vi "EBA Leak test.vi"() -> ()   [LabVIEW 2025]
uses:
  Control EBA.ctl
panel:
  out "Current int":i32
  out "Exit - Entry":i32
  out "Entry int":i32
  out "Exit":i32
  in  "Tab Control":enum32{"Page 1", "Page 2"}(tab)
  out "Checkbox":bool
  out "Save Status":string
  out "Leak rate cc/min":dbl format="%.2f"
  out "Pressure vs Time":dynamicdata(graph)
  out "Info":string
  in  "Stop":bool
  in  "Start":bool
  out "Initial Pressure (Bar)":dbl format="%.3f"
  in  "File Location":path=path "C:/Users/G MOHANASUNDAR/OneDrive/Desktop/Project_EBA/Raw Data/Leak.xlsx" caption="Filename"
  out "Hold Time (s)":dbl format="%.2g"
  out "Current Pressure (Bar)":dbl format="%.2f"
  out "Final Pressure (Bar)":dbl format="%.2f"
  out "error out":errorcluster
  in  "Hold time (s)":dbl=60.0 format="%#_13g"
  # "EBA LEAK THROUGH PUSH TEST"
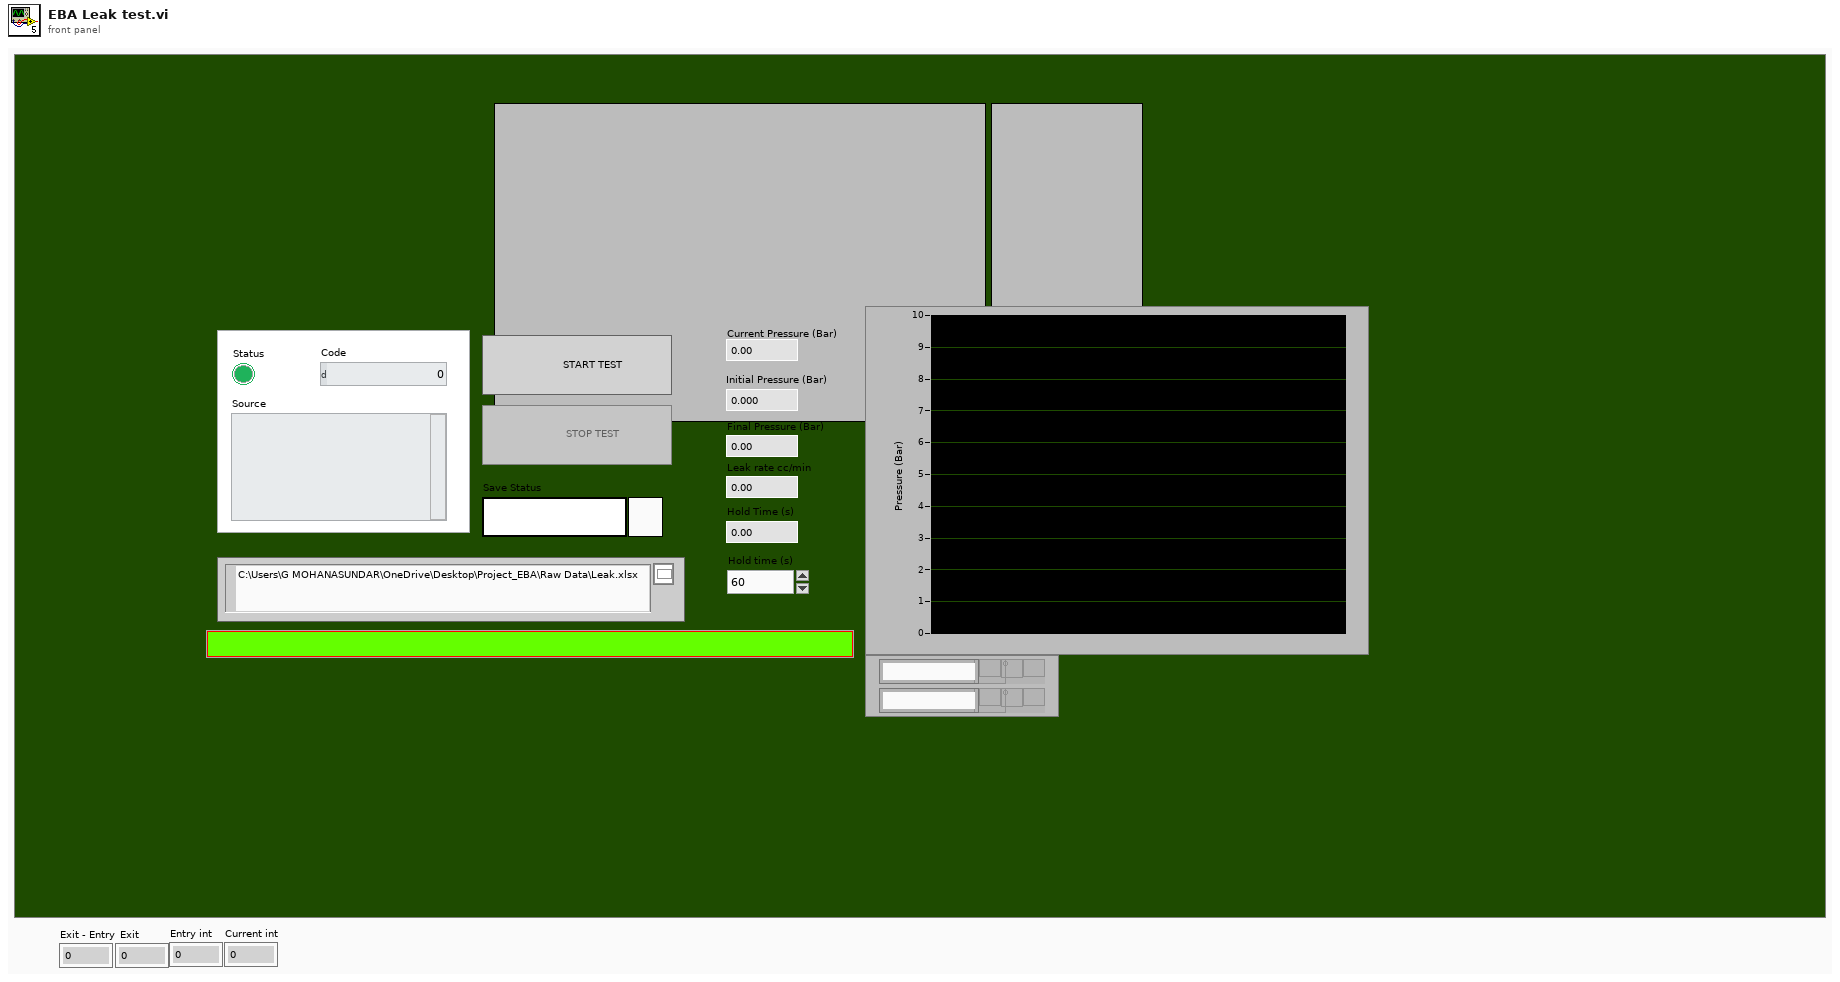
[diagram p1: front panel]
types:
  T1 = typedef "Control EBA.ctl" = enum16{"Wait for event", "Running", "Log", "Stopped", "Leak check", "Calc", "Login", "Update"}
  T2 = cluster{"True?":bool, "time":dbl, "pressure":dbl}
  T3 = enum8{"Enabled", "Disabled", "Disabled and Grayed Out"}
  T4 = enum16{"Wait for event", "Running", "Log", "Stopped"}
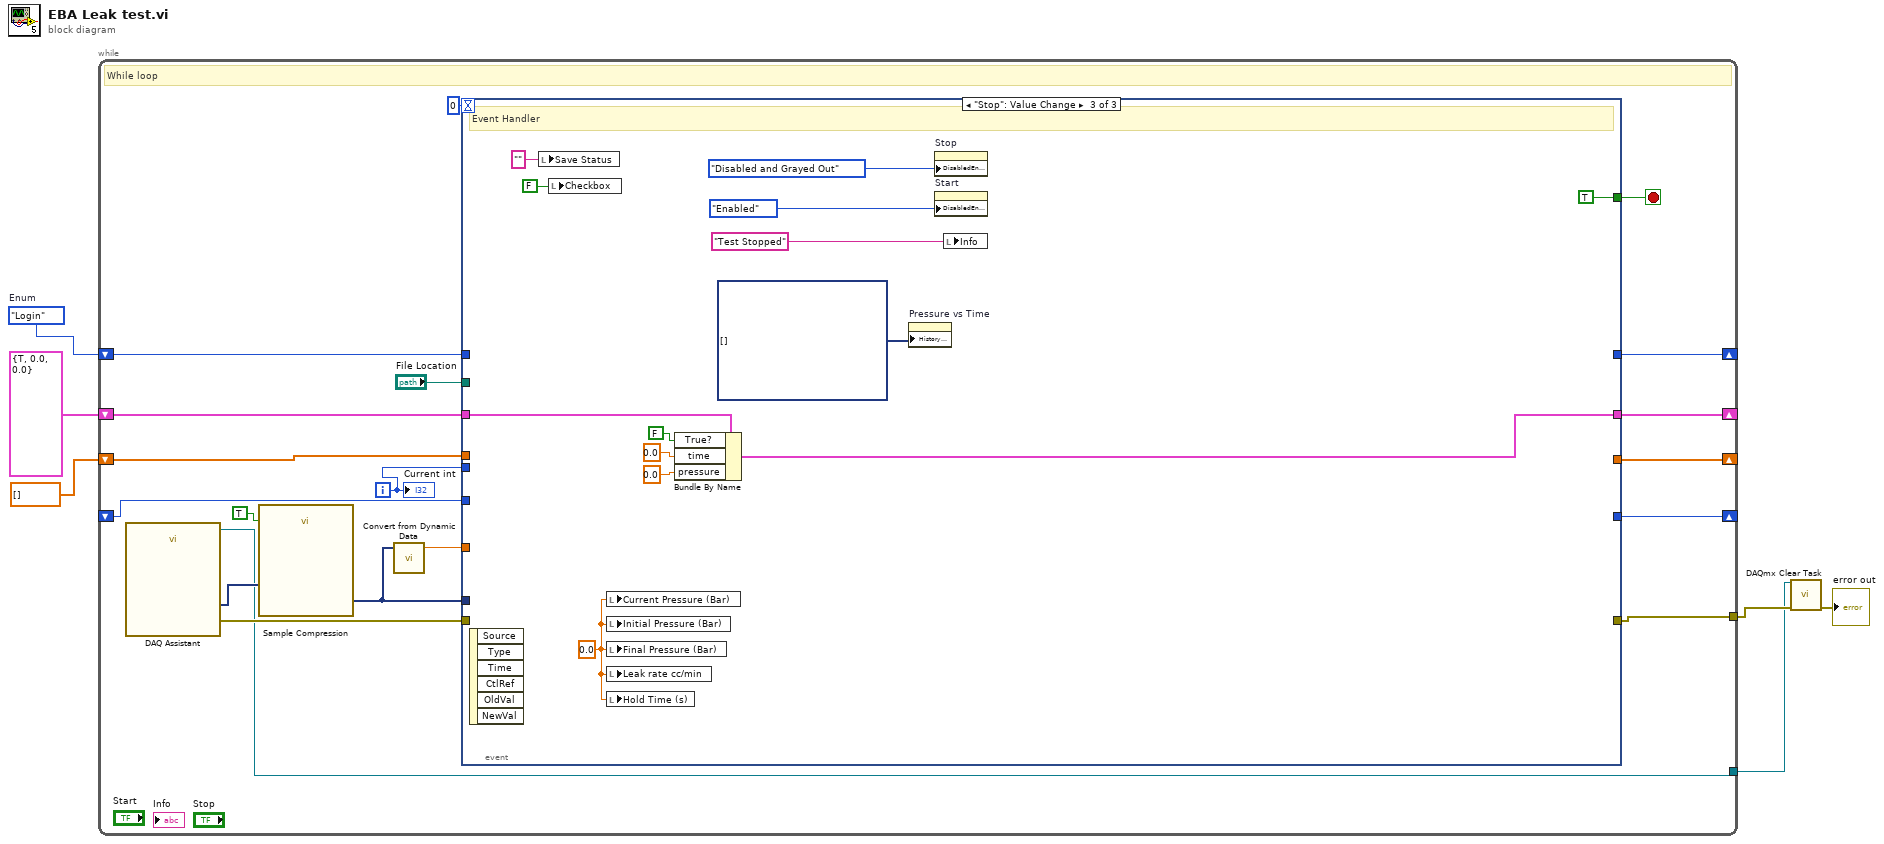
[diagram p0: block diagram]
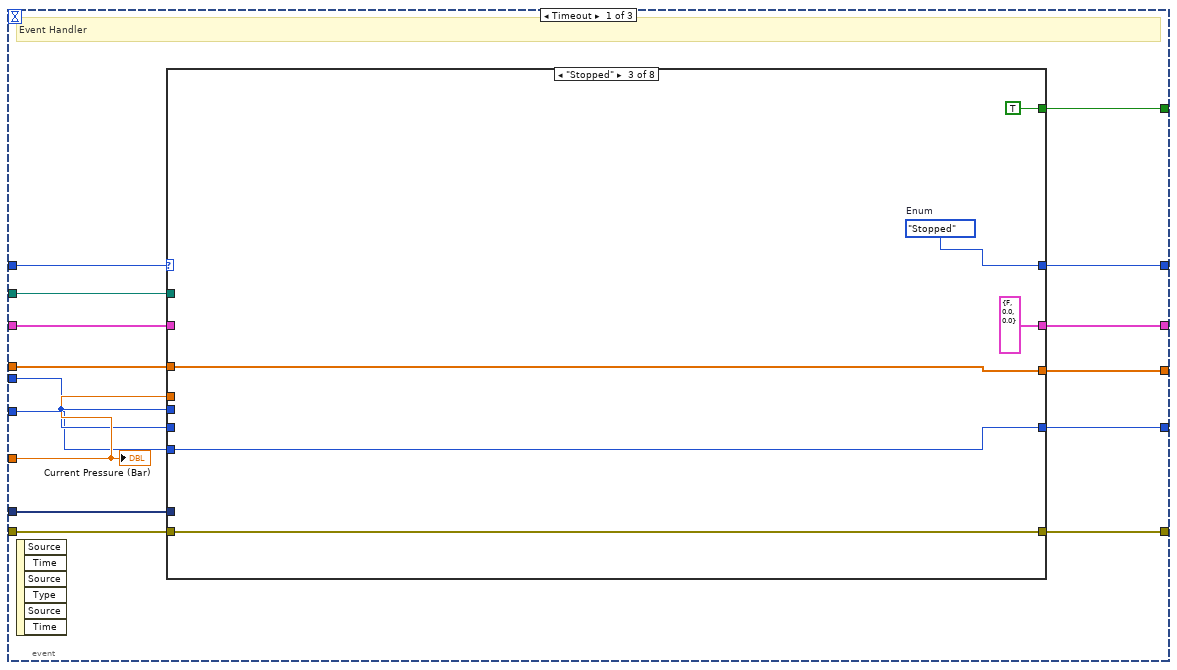
[diagram p2: hidden frame]
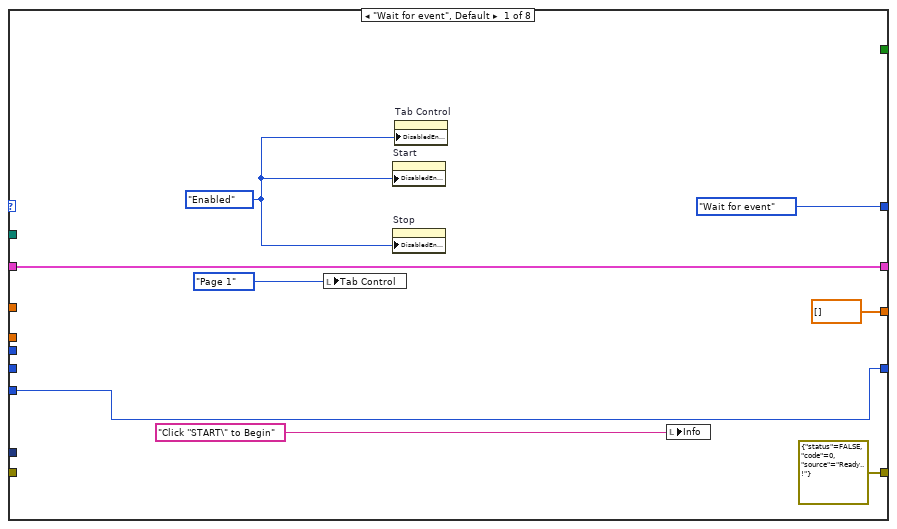
[diagram p3: hidden frame]
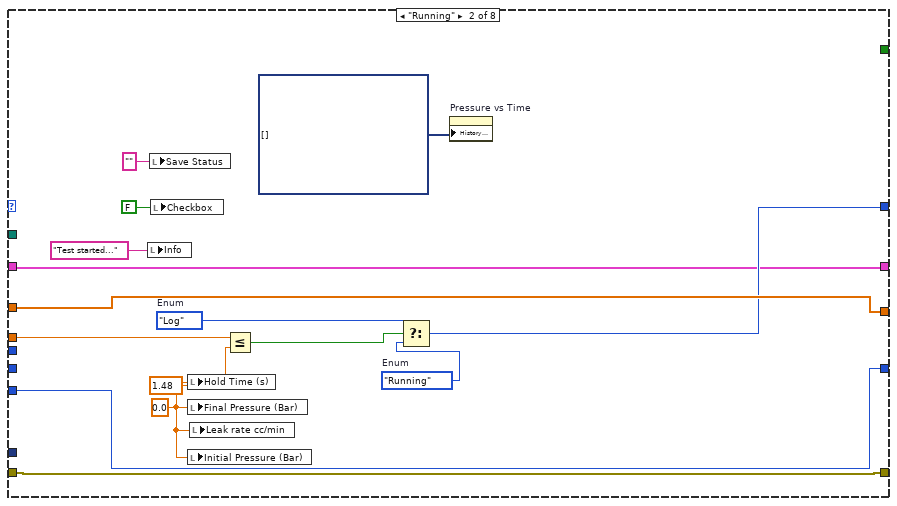
[diagram p4: hidden frame]
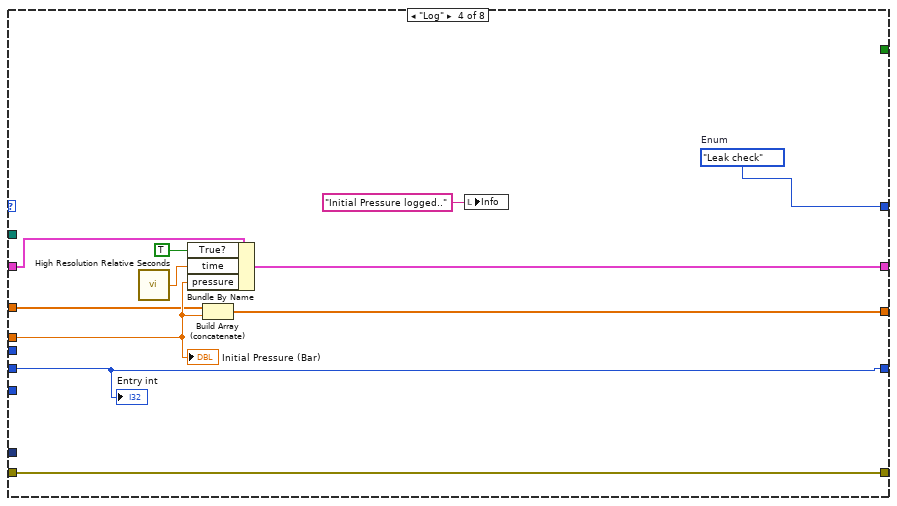
[diagram p5: hidden frame]
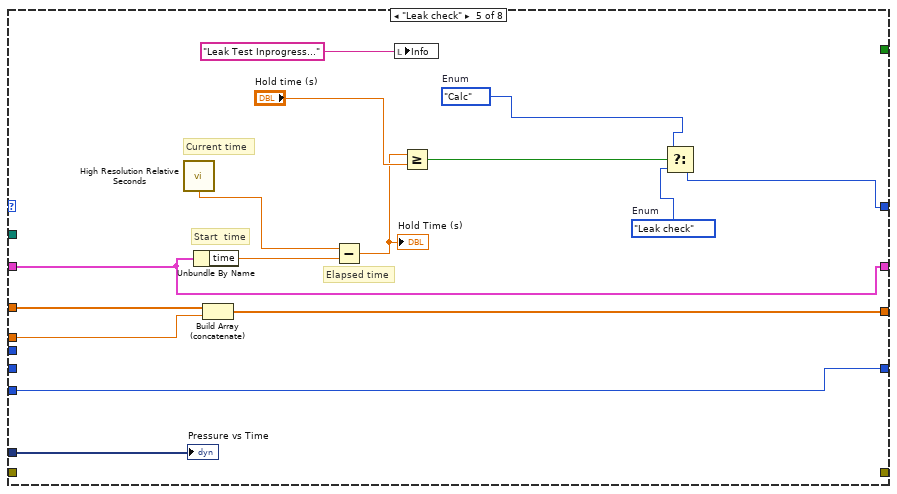
[diagram p6: hidden frame]
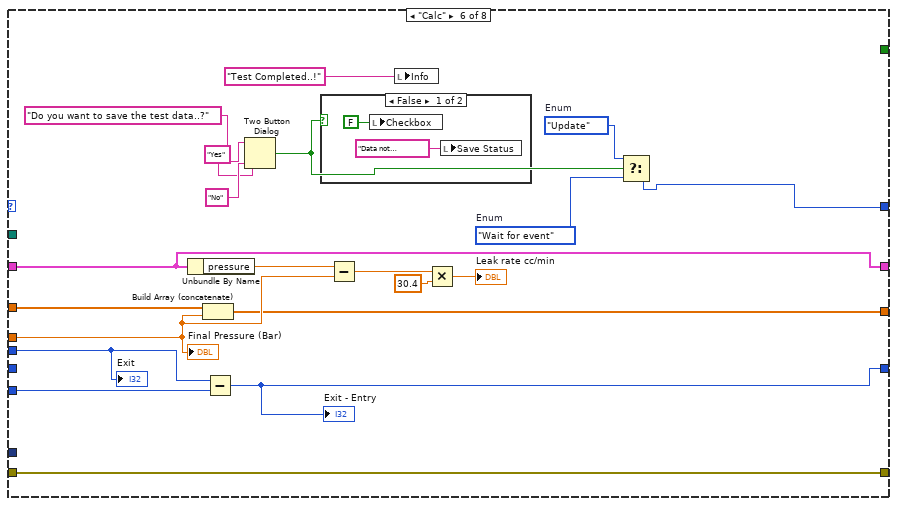
[diagram p7: hidden frame]
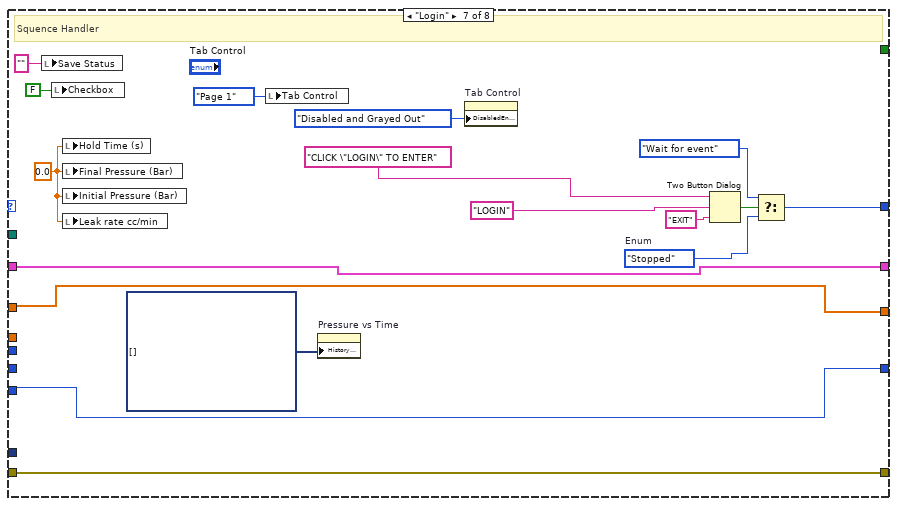
[diagram p9: hidden frame]
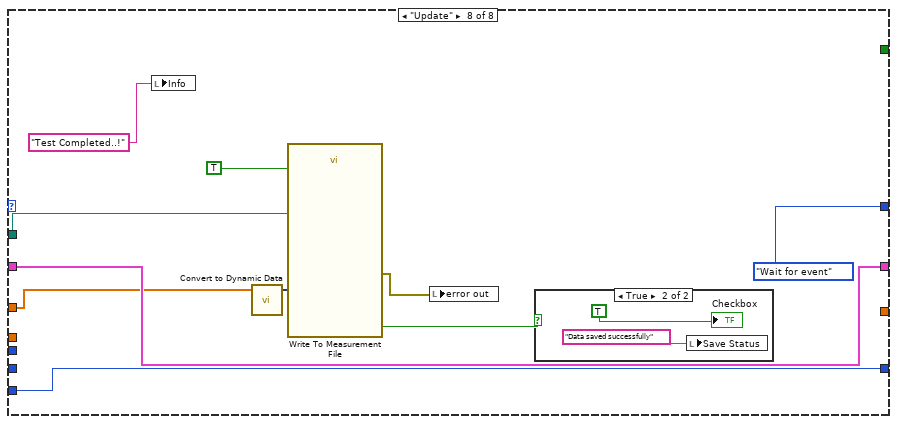
[diagram p10: hidden frame]
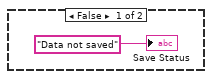
[diagram p11: hidden frame]
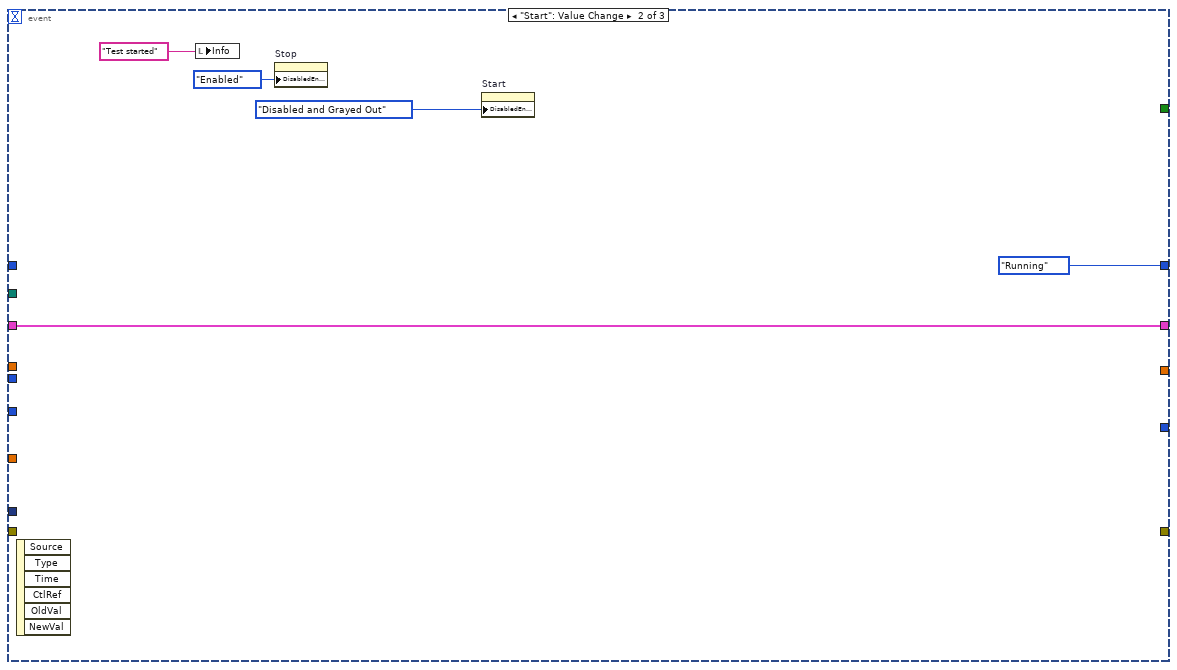
[diagram p12: hidden frame]
diagram:
  w4 = Control_EBA."Login"  # Enum
  n1 = while {
    shift-right: [w23] -> _
    shift-left: T2 {"True?"=TRUE, "time"=0.0, "pressure"=0.0} -> [w24]
    shift-right: [w15] -> _
    shift-left: _ -> [w14]
    shift-right: [w12] -> _
    shift-left: dbl[] [] -> [w13]
    shift-right: [w10] -> _
    shift-left: w4 -> [w25]
    tunnel: [w8] -> w3
    tunnel: [w7] -> w1
    i -> [w16]
    stop <- w22 stop-if-true
    # "While loop"
    n2 = call "DAQ Assistant"() -> ("task out"=w7:refnum<k21>, "data"=w19:dynamicdata, "error out"=w20:errorcluster)  [unwired: 16 in, 1 out]
    n3 = call "Sample Compression"("Enable"=TRUE, "Signals"=w19) -> ("Mean"=w18:dynamicdata)  [unwired: 7 in, 2 out]
    n4 = call "Convert from Dynamic Data"("Dynamic Data Type"=w18) -> ("Scalar"=w21:dbl)  [unwired: 3 in]
    n5 = event shown="[2] \"Stop\": Value Change" {
      selector: _ -> [_ _ _]
      dyn-events: _ -> [_ _ _]
      timeout: 0 -> [_ _ _]
      tunnel: w25 -> [w40 _ _]
      tunnel: w24 -> [w39 w151 w164]
      tunnel: [w38 w151 w163] -> w23
      tunnel: [w27 T4."Running" _] -> w10
      tunnel: [w37 _ TRUE] -> w22
      tunnel: w21 -> [w33 _ _]
      tunnel: [w36 _ _] -> w8
      tunnel: w20 -> [w35 _ _]
      tunnel: w18 -> [w34 _ _]
      tunnel: w16 -> [w31 _ _]
      tunnel: [w32 _ _] -> w15
      tunnel: w14 -> [w30 _ _]
      tunnel: w13 -> [w29 _ _]
      tunnel: [w28 _ _] -> w12
      tunnel: "File Location" -> [w26 _ _]
      event Timeout {
        # "Event Handler"
        n6 = event-data() -> ()  [unwired: 1 in, 6 out]
        n7 = case shown="\"Stopped\"" w40 {
          tunnel: w39 -> [w48 w52 _ w80 w93 w112 w129 w140]
          tunnel: w33 -> [_ w63 _ w72 w84 w105 _ _]
          tunnel: [w48 w52 T2 {"True?"=FALSE, "time"=0.0, "pressure"=0.0} w79 w93 w112 w129 w140] -> w38
          tunnel: [_ _ TRUE _ _ _ _ _] -> w37
          tunnel: [errorcluster {"status"=FALSE, "code"=0, "source"="Ready..!"} ("error out") w60 w67 w76 _ w111 w126 _] -> w36
          tunnel: w35 -> [_ w60 w67 w76 _ w111 w126 _]
          tunnel: w34 -> [_ _ _ _ w85 _ _ _]
          tunnel: w31 -> [_ _ _ w74 _ _ _ _]
          tunnel: [w44 w58 w66 w74 w88 w107 w119 w141] -> w32
          tunnel: w31 -> [_ _ _ _ _ w109 _ _]
          tunnel: w30 -> [w44 w58 w66 _ w88 w108 w119 w141]
          tunnel: w29 -> [_ w57 w65 w71 w87 w106 w118 w136]
          tunnel: [dbl[] [] w57 w65 w73 w86 w104 w118 _] -> w28
          tunnel: [Control_EBA."Wait for event" w54 w64 w70 w81 w102 w124 Control_EBA."Wait for event" ("Enum")] -> w27
          tunnel: w26 -> [_ _ _ _ _ _ _ w143]
          frame "Wait for event", Default {
            w42 = T3."Enabled" ("Disabled")
            n8 = local write "Tab Control"(enum32{"Page 1", "Page 2"}."Page 1" ("Tab Control")) -> ()
            n9 = property on="Start" class="Bool"("DisabledEnum"=w42) -> ()  [unwired: 2 in, 2 out]
            n10 = property on="Stop" class="Bool"("DisabledEnum"=w42) -> ()  [unwired: 2 in, 2 out]
            n11 = property on="Tab Control" class="TabCtl (strict)"("DisabledEnum"=w42) -> ()  [unwired: 2 in, 2 out]
            n12 = local write "Info"("Click ''START\" to Begin" ("Info")) -> ()
          }
          frame "Running" {
            w56 = Control_EBA."Running"  # Enum
            w55 = Control_EBA."Log"  # Enum
            w53 = 0.0 ("Start Pr-0s")
            n13 = local write "Info"("Test started..." ("Info")) -> ()
            n14 = local write "Save Status"("" ("Save Status")) -> ()
            n15 = local write "Checkbox"(FALSE ("Checkbox")) -> ()
            n16 = local write "Hold Time (s)"(w53) -> ()
            n17 = local write "Final Pressure (Bar)"(w53) -> ()
            n18 = local write "Initial Pressure (Bar)"(w53) -> ()
            n19 = local write "Leak rate cc/min"(w53) -> ()
            n20 = Less Or Equal?(x=w63, y=1.48) -> (x <= y?=w61:bool)
            n21 = Select(t=w55, s=w61, f=w56) -> (s? t:f=w54:T1)
            n22 = property on="Pressure vs Time" class="WFChart (strict)"("History Data"=dynamicdata[] []) -> ()  [unwired: 2 in, 2 out]
          }
          frame "Stopped" {
            w64 = Control_EBA."Stopped"  # Enum
          }
          frame "Log" {
            w70 = Control_EBA."Leak check"  # Enum
            n23 = call <vilib>:"High Resolution Relative Seconds.vi"() -> ("relative seconds"=w78:dbl)
            n24 = Bundle By Name(cluster=w80, "True?"=TRUE, "time"=w78, "pressure"=w72) -> (w79:T2)
            n25 = Build Array (concatenate)(w71, w72) -> (w73:dbl[])
            n26 = local write "Info"("Initial Pressure logged.." ("Info")) -> ()
            "Initial Pressure (Bar)" <- w72
            "Entry int" <- w74
          }
          frame "Leak check" {
            w83 = Control_EBA."Calc"  # Enum
            w82 = Control_EBA."Leak check"  # Enum
            # "Start  time"
            # "Current time"
            # "Elapsed time"
            n27 = call <vilib>:"High Resolution Relative Seconds.vi"() -> ("relative seconds"=w94:dbl)
            n28 = Unbundle By Name(w93) -> ("time"=w95:dbl)
            n29 = Build Array (concatenate)(w87, w84) -> (w86:dbl[])
            n30 = Subtract(x=w94, y=w95) -> (x-y=w90:dbl)
            "Hold Time (s)" <- w90
            n31 = local write "Info"("Leak Test Inprogress..." ("Info")) -> ()
            n32 = Greater Or Equal?(x=w90, y="Hold time (s)") -> (x >= y?=w91:bool)
            n33 = Select(t=w83, s=w91, f=w82) -> (s? t:f=w81:T1)
            "Pressure vs Time" <- w85
          }
          frame "Calc" {
            w100 = Control_EBA."Wait for event"  # Enum
            w101 = Control_EBA."Update"  # Enum
            n34 = Unbundle By Name(w112) -> ("pressure"=w115:dbl)
            n35 = Build Array (concatenate)(w106, w105) -> (w104:dbl[])
            n36 = Subtract(x=w109, y=w108) -> (x-y=w107:i32)
            "Exit - Entry" <- w107
            n37 = Two Button Dialog(message="Do you want to save the test data..?", 1:"No" ("F button name (\"Cancel\")"), 2:"Yes" ("T button name (\"OK\")")) -> (T button?=w96:bool)
            n38 = case shown="False" w96 {
              frame False {
                n39 = local write "Checkbox"(FALSE ("Checkbox")) -> ()
                n40 = local write "Save Status"("Data not                     saved " ("Save Status")) -> ()
              }
              frame True {
              }
            }
            n41 = Subtract(x=w115, y=w105) -> (x-y=w114:dbl)
            n42 = local write "Info"("Test Completed..!" ("Info")) -> ()
            n43 = Multiply(x=w114, y=30.4) -> (x*y=→"Leak rate cc/min":dbl)
            n44 = Select(t=w101, s=w96, f=w100) -> (s? t:f=w102:T1)
            "Final Pressure (Bar)" <- w105
            "Exit" <- w109
          }
          frame "Login" {
            w121 = 0.0 ("Start Pr-0s")
            w125 = Control_EBA."Stopped"  # Enum
            # "Squence Handler"
            n45 = local write "Save Status"("" ("Save Status")) -> ()
            n46 = local write "Checkbox"(FALSE ("Checkbox")) -> ()
            n47 = local write "Hold Time (s)"(w121) -> ()
            n48 = local write "Final Pressure (Bar)"(w121) -> ()
            n49 = local write "Initial Pressure (Bar)"(w121) -> ()
            n50 = local write "Leak rate cc/min"(w121) -> ()
            n51 = local write "Tab Control"(enum32{"Page 1", "Page 2"}."Page 1" ("Tab Control")) -> ()
            n52 = property on="Pressure vs Time" class="WFChart (strict)"("History Data"=dynamicdata[] []) -> ()  [unwired: 2 in, 2 out]
            n53 = property on="Tab Control" class="TabCtl (strict)"("DisabledEnum"=T3."Disabled and Grayed Out" ("Disabled")) -> ()  [unwired: 2 in, 2 out]
            n54 = Two Button Dialog(message="CLICK \"LOGIN\" TO ENTER", 1:"EXIT" ("F button name (\"Cancel\")"), 2:"LOGIN" ("T button name (\"OK\")")) -> (T button?=w131:bool)
            n55 = Select(t=Control_EBA."Wait for event", s=w131, f=w125) -> (s? t:f=w124:T1)
          }
          frame "Update" {
            n56 = local write "Info"("Test Completed..!" ("Info")) -> ()
            n57 = call "Convert to Dynamic Data"("Array"=w136) -> ("Dynamic Data Type"=w135:dynamicdata)  [unwired: 3 in]
            n58 = call "Write To Measurement File"("Signals"=w135, "Enable"=TRUE, "Filename"=w143) -> ("Saving Data"=w138:bool, "error out"=w144:errorcluster)  [unwired: 14 in, 1 out]
            n59 = local write "error out"(w144) -> ()
            n60 = case shown="True" w138 {
              frame False {
                "Save Status" <- "Data not saved" ("Save Status")
              }
              frame True {
                n61 = local write "Save Status"("Data saved successfully" ("Save Status")) -> ()
                "Checkbox" <- TRUE ("Checkbox")
              }
            }
          }
        }
        "Current Pressure (Bar)" <- w33
      }
      event "Start": Value Change {
        n62 = event-data() -> ()  [unwired: 1 in, 6 out]
        n63 = local write "Info"("Test started" ("Info")) -> ()
        n64 = property on="Stop" class="Bool"("DisabledEnum"=T3."Enabled" ("Disabled")) -> ()  [unwired: 2 in, 2 out]
        n65 = property on="Start" class="Bool"("DisabledEnum"=T3."Disabled and Grayed Out" ("Disabled")) -> ()  [unwired: 2 in, 2 out]
      }
      event "Stop": Value Change {
        w153 = 0.0 ("Start Pr-0s")
        # "Event Handler"
        n66 = event-data() -> ()  [unwired: 1 in, 6 out]
        n67 = local write "Save Status"("" ("Save Status")) -> ()
        n68 = local write "Checkbox"(FALSE ("Checkbox")) -> ()
        n69 = local write "Current Pressure (Bar)"(w153) -> ()
        n70 = local write "Initial Pressure (Bar)"(w153) -> ()
        n71 = local write "Final Pressure (Bar)"(w153) -> ()
        n72 = local write "Leak rate cc/min"(w153) -> ()
        n73 = local write "Hold Time (s)"(w153) -> ()
        n74 = Bundle By Name(cluster=w164, "True?"=FALSE, "time"=0.0, "pressure"=0.0) -> (w163:T2)
        n75 = property on="Pressure vs Time" class="WFChart (strict)"("History Data"=dynamicdata[] []) -> ()  [unwired: 2 in, 2 out]
        n76 = property on="Stop" class="Bool"("DisabledEnum"=T3."Disabled and Grayed Out" ("Disabled")) -> ()  [unwired: 2 in, 2 out]
        n77 = property on="Start" class="Bool"("DisabledEnum"=T3."Enabled" ("Disabled")) -> ()  [unwired: 2 in, 2 out]
        n78 = local write "Info"("Test Stopped" ("Info")) -> ()
      }
    }
    "Current int" <- w16
  }
  n79 = call <vilib>:"DAQmx Clear Task.vi"("task in"=w1, "error in"=w3) -> ("error out"=→"error out":errorcluster)  [unwired: 13 in]
